vi "CalculoRampaDescida.vi"(8 "TempoRampa":dbl, 9 "PicoMax":dbl, 10 "CiclosIn":i32, 11 "OndaIn":cluster{"X":dbl, "Y":dbl}[](array[cluster])) -> (2 "CiclosOut":i32, 3 "OndaOut":cluster{"X":dbl, "Y":dbl}[](graph))   [LabVIEW 2019]
panel:
  # "segundos"
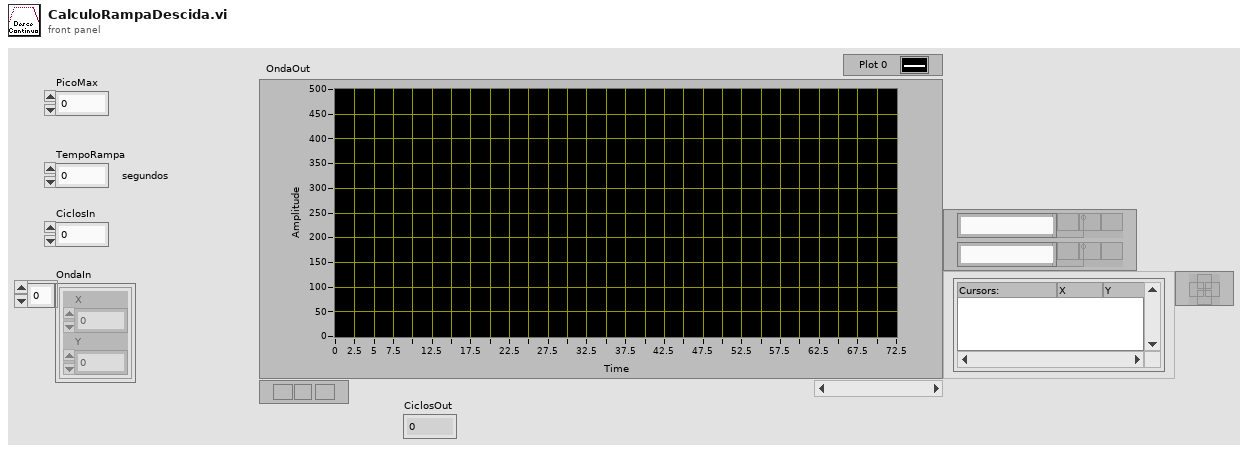
[diagram p1: front panel]
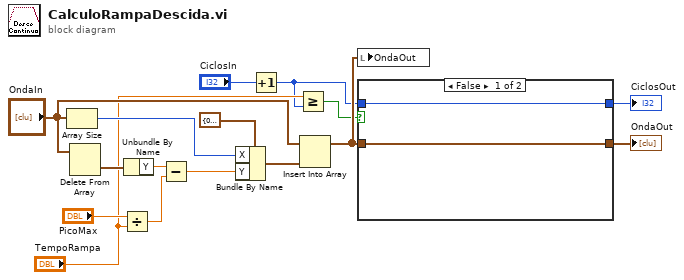
[diagram p0: block diagram]
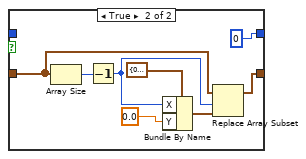
[diagram p2: hidden frame]
diagram:
  n1 = Array Size(array="OndaIn") -> (size(s)=w14:i32)
  n2 = Delete From Array(array="OndaIn") -> (deleted portion=w9:cluster{"X":dbl, "Y":dbl})  [unwired: 2 in, 1 out]
  n3 = Divide(x="PicoMax", y="TempoRampa") -> (x/y=w11:dbl)
  n4 = Unbundle By Name(w9) -> ("Y"=w8:dbl)
  n5 = Subtract(x=w8, y=w11) -> (x-y=w10:dbl)
  n6 = Bundle By Name(cluster=cluster{"X":dbl, "Y":dbl} {"X"=0.0, "Y"=0.0} ("new element/subarray"), "X"=w14, "Y"=w10) -> (w12:cluster{"X":dbl, "Y":dbl})
  n7 = Increment(x="CiclosIn") -> (x+1=w2:i32)
  n8 = Greater Or Equal?(x="TempoRampa", y=w2) -> (x >= y?=w4:bool)
  n9 = Insert Into Array(array="OndaIn", new element=w12) -> (w15:cluster{"X":dbl, "Y":dbl}[])  [unwired: 1 in]
  n10 = local write "OndaOut"(w15) -> ()
  n11 = case shown="False" w4 {
    tunnel: w15 -> [w17 w26]
    tunnel: [w18 0] -> w3
    tunnel: w2 -> [w18 _]
    tunnel: [w17 w24] -> w1
    frame False {
    }
    frame True {
      n12 = Array Size(array=w26) -> (size(s)=w23:i32)
      n13 = Decrement(x=w23) -> (x-1=w19:i32)
      n14 = Bundle By Name(cluster=cluster{"X":dbl, "Y":dbl} {"X"=0.0, "Y"=0.0} ("new element/subarray"), "X"=w19, "Y"=0.0) -> (w20:cluster{"X":dbl, "Y":dbl})
      n15 = Replace Array Subset(array=w26, new element=w20, index=w19) -> (w24:cluster{"X":dbl, "Y":dbl}[])
    }
  }
  "CiclosOut" <- w3
  "OndaOut" <- w1
